vi "GetFormattedValue.vi"(8 "error in (no error)":errorcluster, 10 "lookup string":string, 11 "property object in":refnum<k7>) -> (0 "error out":errorcluster, 2 "value":string, 3 "property object out":refnum<k7>)   [LabVIEW 2019]
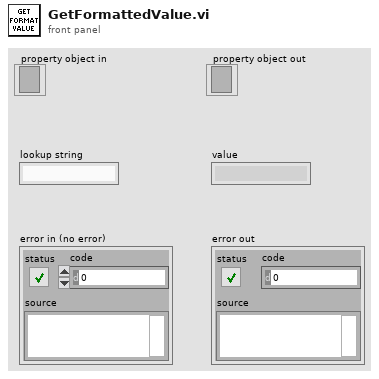
[diagram p1: front panel]
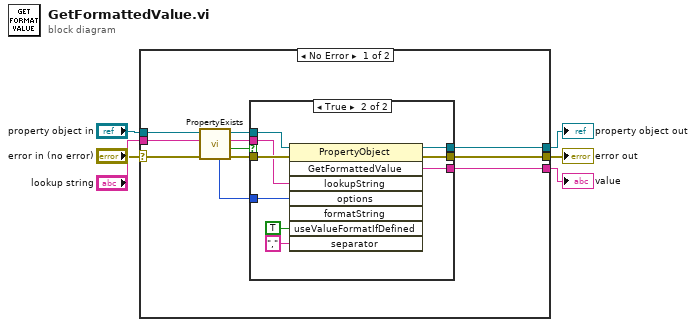
[diagram p0: block diagram]
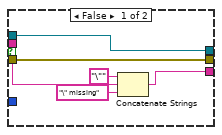
[diagram p2: hidden frame]
diagram:
  n1 = case shown="No Error" "error in (no error)" {
    selector: "error in (no error)" -> [w10 w33]
    tunnel: [w17 w34] -> w6
    tunnel: [w16 w33] -> w5
    tunnel: "lookup string" -> [w13 _]
    tunnel: "property object in" -> [w11 w34]
    tunnel: [w9 _] -> w1
    frame No Error {
      n2 = call "PropertyExists.vi"("error in (no error)"=w10, "lookup string in"=w13, "property object in"=w11) -> ("error out"=w14:errorcluster, "exists"=w15:bool, "lookup string out"=w8:string, "property object out"=w12:refnum<k7>, "options"=w7:i32)  [unwired: 4 in]
      n3 = case shown="True" w15 {
        tunnel: w12 -> [w18 w31]
        tunnel: w8 -> [w23 w30]
        tunnel: w14 -> [w19 w32]
        tunnel: [w20 w27] -> w9
        tunnel: [w19 w26] -> w16
        tunnel: [w18 w25] -> w17
        tunnel: w7 -> [_ w24]
        frame False {
          n4 = Concatenate Strings("\"" ("string"), w23, "\" missing" ("string")) -> (w20:string)
        }
        frame True {
          n5 = invoke class="PropertyObject" method="GetFormattedValue"(reference=w31, error in=w32, "lookupString"=w30, "options"=w24, "useValueFormatIfDefined"=TRUE, "separator"=",") -> (reference out=w25:refnum<k7>, error out=w26:errorcluster, "GetFormattedValue"=w27:string)  [unwired: 2 in, 5 out]
        }
      }
    }
    frame Error {
    }
  }
  "property object out" <- w6
  "error out" <- w5
  "value" <- w1
